vi "ServerProcess.vi"(0 "occurrence":refnum<k4>, 1 "TCP port":u16=62001, 5 "error in (no error)":errorcluster) -> (19 "error out":errorcluster)   [LabVIEW 2017, in "G#DebugServer.lvclass"]
doc: "Server process on the remote target."
uses:
  G#DebugServer.lvclass
  utils/LocalProcessData.ctl
  utils/TCPCommand.ctl
  G#Object/utils/G#Object_Event.ctl
  G#Object/utils/G#Object_EventType.ctl
  G#Object/utils/G#Object_ObjectInfoType.ctl
  G#Object/utils/G#Object_CreateMethod.ctl
  G#Object/G#Object.lvclass
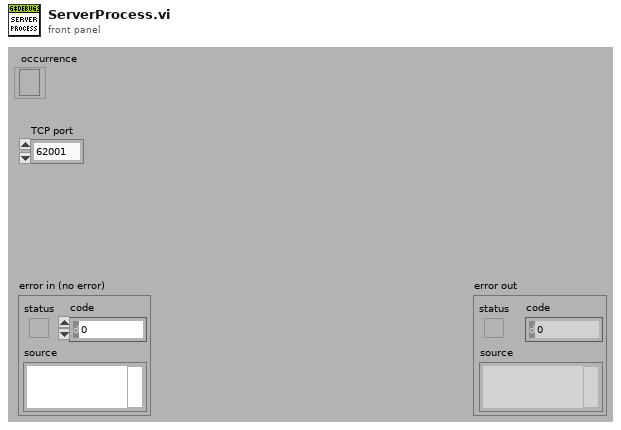
[diagram p1: front panel]
types:
  T1 = cluster{"ClientAddress":u32, "G#Event":refnum<user-event>, "CreatedG#event?":bool, "ConnectionID":refnum<k5>, "Enabled":bool}
  T2 = typedef "G#Object.lvclass/G#Object_Event.ctl" = cluster{"EventType":T3, "ObjectInfo":T4, "Ref":refnum<class "G#Object.lvclass">, "Time Stamp":timestamp, "LogText":string, "Parameters":variant[]}
  T3 = typedef "G#Object.lvclass/G#Object_EventType.ctl" = enum16{"Created new", "Looked up existing", "Deleted", "Forced delete", "Not deleted", "Garbage collected", "Cleared", "User", "Error", "External create object", "External create class attributes", "Created class attributes", "Run constructor", "Run constructor done", "Run open method", "Run open method done"}
  T4 = typedef "G#Object.lvclass/G#Object_ObjectInfoType.ctl" = cluster{"ObjectName":string, "ObjectID":u32, "Users":i32, "Counter":bool, "AttributeRefs":u32[], "FullClassName":string, "ClassName":string, "CreateMethod":T5, "GenericDestructorExists":bool, "Owner":string}
  T5 = typedef "G#Object.lvclass/G#Object_CreateMethod.ctl" = enum16{"Create", "Create or look up existing", "Look up existing"}
  T6 = typedef "G#DebugServer.lvclass/LocalProcessData.ctl" = cluster{"Event":string, "Command":T7, "Data":string, "Address":u32}
  T7 = typedef "G#DebugServer.lvclass/TCPCommand.ctl" = u8
  T8 = typedef "G#Object.lvclass/G#Object_ClassHierarchy.ctl" = cluster{"ClassName":string, "FullClassName":string, "ClassPath":path, "IsLeaf":bool}
  T9 = typedef "G#Object.lvclass/G#Object_ClassInfoType.ctl" = cluster{"ClassName":string, "ObjectInfo":T4[], "ObjectRefs":refnum<class "G#Object.lvclass">[], "TypeRef":refnum<class "G#Object.lvclass">}
  T10 = cluster{"G#DebugServer ref":refnum<class "G#Object.lvclass">, "attributes":variant[]}
  T11 = cluster{"G#DebugServer ref":refnum<class "G#Object.lvclass">, "class attributes":variant[]}
  T12 = cluster{"G#DebugServer ref":refnum<class "G#Object.lvclass">, "string":string}
  T13 = cluster{"G#DebugServer ref":refnum<class "G#Object.lvclass">, "class hierarchy":T8[]}
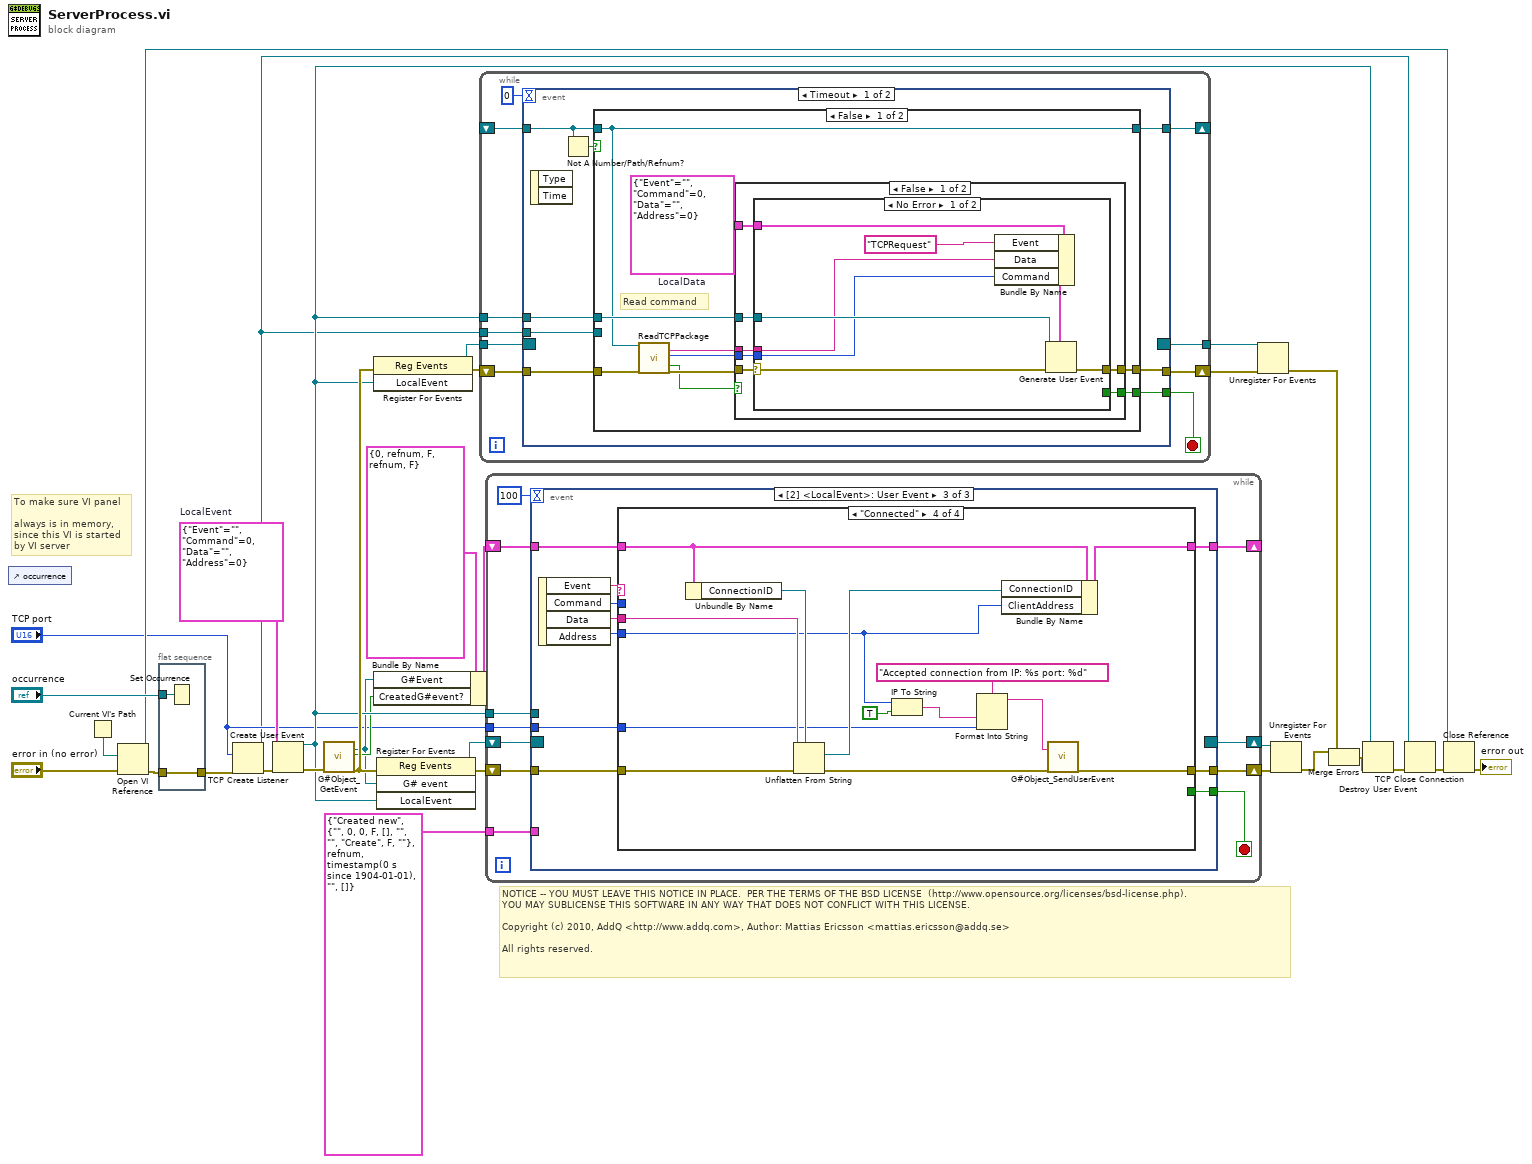
[diagram p0: block diagram]
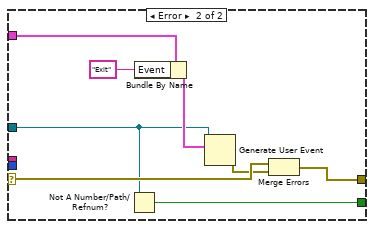
[diagram p2: hidden frame]
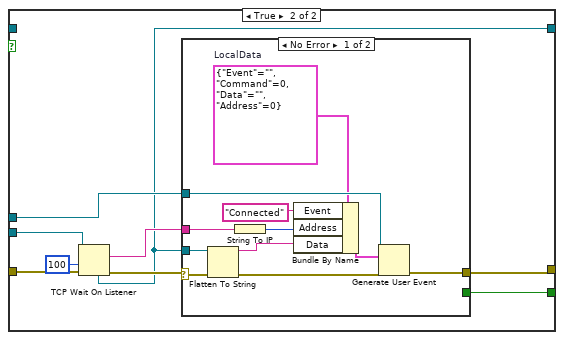
[diagram p4: hidden frame]
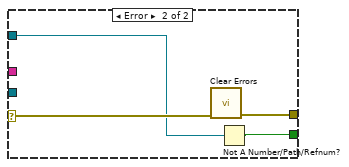
[diagram p5: hidden frame]
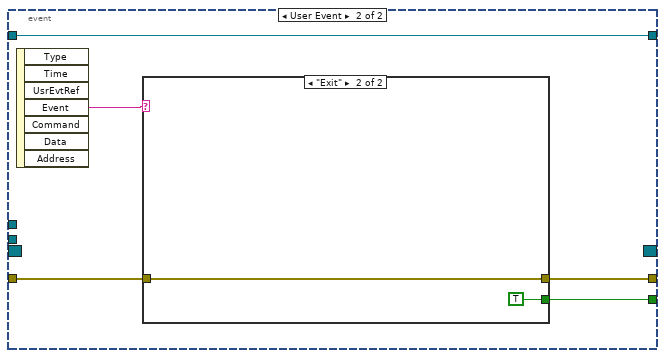
[diagram p6: hidden frame]
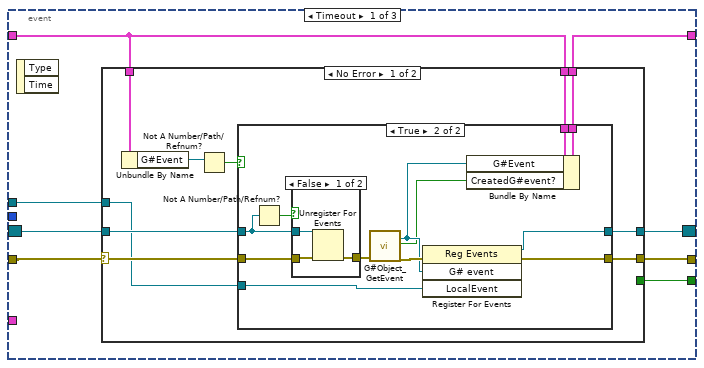
[diagram p8: hidden frame]
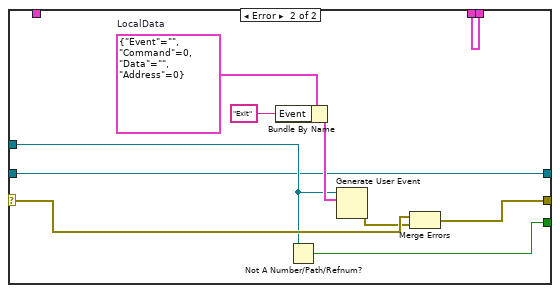
[diagram p11: hidden frame]
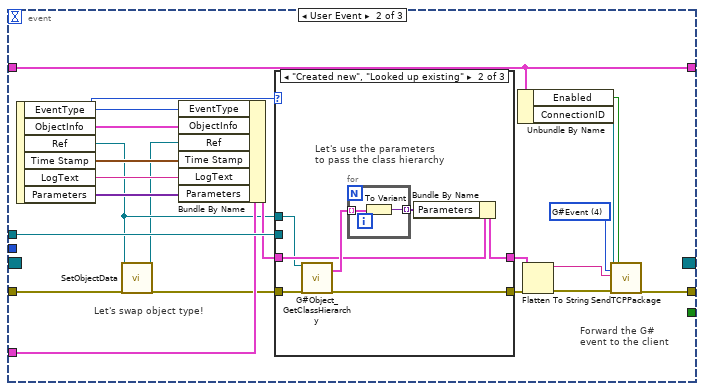
[diagram p12: hidden frame]
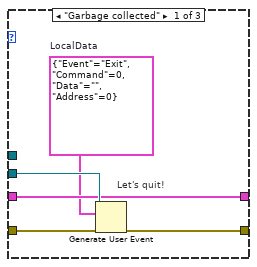
[diagram p13: hidden frame]
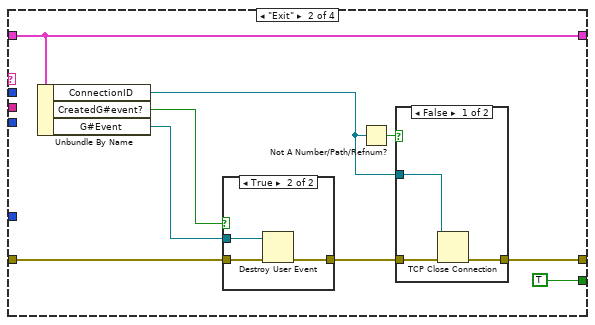
[diagram p16: hidden frame]
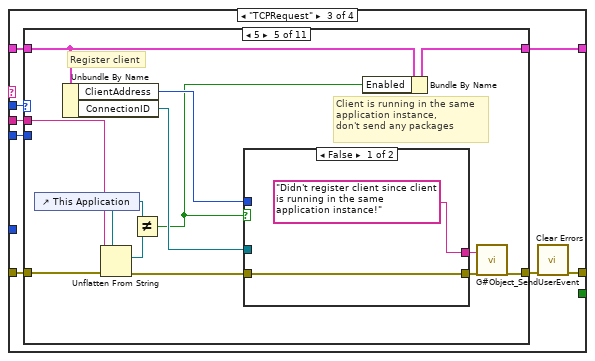
[diagram p19: hidden frame]
diagram:
  w13 = T6 {"Event"="", "Command"=0, "Data"="", "Address"=0}  # LocalEvent
  # "NOTICE -- YOU MUST LEAVE THIS NOTICE IN PLACE.  PER THE TERMS OF THE BSD LICENSE  (http://www.opensource.org/licenses/bsd-license.php).\nYOU MAY SUBLICENSE THIS SOFTWARE IN ANY WAY THAT DOES NOT CONFLICT WITH THIS LICENSE.\n\nCopyright (c) 2010, AddQ <http://www.addq.com>, Author: Mattias Ericsson <mattias.ericsson@addq.se>\n\nAll rights reserved."
  # "To make sure VI panel\n\nalways is in memory,\nsince this VI is started\nby VI server"
  n1 = control-ref of="occurrence"() -> ()  [unwired: 1 out]
  n2 = Current VI's Path() -> (path=w32:path)
  n3 = Open VI Reference(vi path=w32, error in (no error)="error in (no error)") -> (vi reference=w27:refnum<vi>, error out=w30:errorcluster)  [unwired: 4 in]
  n4 = flat-sequence {
    tunnel: "occurrence" -> [w34]
    tunnel: w30 -> [w33]
    tunnel: [w33] -> w6
    frame #0 {
      n5 = Set Occurrence(w34) -> ()
    }
  }
  n6 = TCP Create Listener(8:w6, 10:"TCP port") -> (0:w5:errorcluster, 3:w1:refnum<k5>)  [unwired: 3 in, 1 out]
  n7 = Create User Event(user event datatype=w13, error in=w5) -> (user event=w12:refnum<user-event>, error out=w15:errorcluster)
  n8 = call "G#Object_GetEvent.vi"("error in (no error)"=w15) -> ("G# event"=w7:refnum<user-event>, "created new"=w8:bool, "error out"=w14:errorcluster)  [unwired: 14 in, 2 out]
  n9 = register-events(error in=w14, w12) -> (reference out=w17:refnum<event-registration>, error out=w22:errorcluster)  [unwired: 1 in]
  n10 = Bundle By Name(cluster=T1 {"ClientAddress"=0, "G#Event"=refnum, "CreatedG#event?"=FALSE, "ConnectionID"=refnum, "Enabled"=FALSE}, "G#Event"=w7, "CreatedG#event?"=w8) -> (w9:T1)
  n11 = register-events(error in=w14, w7, w12) -> (reference out=w25:refnum<event-registration>, error out=w26:errorcluster)  [unwired: 1 in]
  n12 = while {
    shift-right: [w41] -> w21
    shift-left: w22 -> [w42]
    tunnel: [w44] -> w20
    tunnel: w17 -> [w43]
    tunnel: w1 -> [w40]
    tunnel: w12 -> [w37]
    shift-right: [w36] -> _
    shift-left: _ -> [w35]
    stop <- w39 stop-if-true
    n13 = event shown="[0] Timeout" {
      selector: w43 -> [_ _]
      dyn-events: [_ _] -> w44
      timeout: 0 -> [_ _]
      tunnel: w42 -> [w50 w115]
      tunnel: [w51 w114] -> w41
      tunnel: w40 -> [w48 _]
      tunnel: [w49 w113] -> w39
      tunnel: w37 -> [w52 _]
      tunnel: [w47 w111] -> w36
      tunnel: w35 -> [w45 w111]
      event Timeout {
        n14 = event-data() -> ()  [unwired: 1 in, 2 out]
        n15 = Not A Number/Path/Refnum?(number/path/refnum=w45) -> (NaN/Path/Refnum?=w46:bool)
        n16 = case shown="False" w46 {
          tunnel: w52 -> [w62 w90]
          tunnel: [w61 w92] -> w51
          tunnel: w50 -> [w59 w95]
          tunnel: [w54 w89] -> w49
          tunnel: w48 -> [_ w94]
          tunnel: [w53 w87] -> w47
          tunnel: w45 -> [w53 _]
          frame False {
            w60 = T6 {"Event"="", "Command"=0, "Data"="", "Address"=0}  # LocalData
            # "Read command"
            n17 = call "ReadTCPPackage.vi"("connection ID"=w53, "error in (no error)"=w59) -> ("payload"=w56:string, "command"=w55:T7, "timeout"=w57:bool, "error out"=w58:errorcluster)  [unwired: 14 in]
            n18 = case shown="False" w57 {
              tunnel: w58 -> [w69 w86]
              tunnel: [w67 w86] -> w61
              tunnel: w62 -> [w68 _]
              tunnel: w60 -> [w66 _]
              tunnel: w56 -> [w65 _]
              tunnel: w55 -> [w64 _]
              tunnel: [w63 _] -> w54
              frame False {
                n19 = case shown="No Error" w69 {
                  selector: w69 -> [w72 w84]
                  tunnel: w68 -> [w77 w79]
                  tunnel: [w76 w85] -> w67
                  tunnel: w66 -> [w75 w82]
                  tunnel: w65 -> [w71 _]
                  tunnel: w64 -> [w70 _]
                  tunnel: [_ w78] -> w63
                  frame No Error {
                    n20 = Bundle By Name(cluster=w75, "Event"="TCPRequest" ("Command"), "Data"=w71, "Command"=w70) -> (w74:T6)
                    n21 = Generate User Event(user event=w77, event data cluster=w74, error in=w72) -> (error out=w76:errorcluster)  [unwired: 1 in, 1 out]
                  }
                  frame Error {
                    n22 = Not A Number/Path/Refnum?(number/path/refnum=w79) -> (NaN/Path/Refnum?=w78:bool)
                    n23 = Bundle By Name(cluster=w82, "Event"="Exit" ("Command")) -> (w81:T6)
                    n24 = Generate User Event(user event=w79, event data cluster=w81) -> (error out=w83:errorcluster)  [unwired: 2 in, 1 out]
                    n25 = Merge Errors(w84, w83) -> (w85:errorcluster)
                  }
                }
              }
              frame True {
                # "Timeout"
              }
            }
          }
          frame True {
            n26 = TCP Wait On Listener(8:w95, 9:100 ("timeout ms (wait forever: -1)"), 11:w94) -> (0:w91:errorcluster, 2:w88:string, 4:w87:refnum<k5>)  [unwired: 1 in, 2 out]
            n27 = case shown="No Error" w91 {
              selector: w91 -> [w100 w109]
              tunnel: [w106 w110] -> w92
              tunnel: w90 -> [w105 w108]
              tunnel: [_ w107] -> w89
              tunnel: w88 -> [w101 _]
              tunnel: w87 -> [w98 _]
              frame No Error {
                w104 = T6 {"Event"="", "Command"=0, "Data"="", "Address"=0}  # LocalData
                n28 = Flatten To String(anything=w98, error in (no error)=w100) -> (data string=w97:string, error out=w99:errorcluster)  [unwired: 2 in, 1 out]
                n29 = String To IP(1:w101) -> (0:w102:u32)
                n30 = Bundle By Name(cluster=w104, "Event"="Connected", "Address"=w102, "Data"=w97) -> (w103:T6)
                n31 = Generate User Event(user event=w105, event data cluster=w103, error in=w99) -> (error out=w106:errorcluster)  [unwired: 1 in, 1 out]
              }
              frame Error {
                n32 = call <vilib>:"Clear Errors.vi"("error in (no error)"=w109) -> ("error out"=w110:errorcluster)  [unwired: 5 in, 1 out]
                n33 = Not A Number/Path/Refnum?(number/path/refnum=w108) -> (NaN/Path/Refnum?=w107:bool)
              }
            }
          }
        }
      }
      event User Event {
        n34 = event-data() -> ("Event"=w112:string)  [unwired: 1 in, 6 out]
        n35 = case shown="\"Exit\"" w112 {
          tunnel: w115 -> [w116 w117]
          tunnel: [w116 w117] -> w114
          tunnel: [_ TRUE] -> w113
          frame Default {
          }
          frame "Exit" {
          }
        }
      }
    }
  }
  n36 = while {
    shift-right: [w126] -> w24
    shift-left: w26 -> [w127]
    tunnel: w12 -> [w124]
    tunnel: T2 {"EventType"=enum."Created new", "ObjectInfo"={"ObjectName"="", "ObjectID"=0, "Users"=0, "Counter"=FALSE, "AttributeRefs"=[], "FullClassName"="", "ClassName"="", "CreateMethod"=enum."Create", "GenericDestructorExists"=FALSE, "Owner"=""}, "Ref"=refnum, "Time Stamp"=timestamp(0 s since 1904-01-01), "LogText"="", "Parameters"=[]} ("G#Event") -> [w122]
    shift-right: [w121] -> _
    shift-left: w9 -> [w120]
    shift-right: [w128] -> w23
    shift-left: w25 -> [w129]
    tunnel: "TCP port" -> [w119]
    stop <- w125 stop-if-true
    n37 = event shown="[2] <LocalEvent>: User Event" {
      selector: w129 -> [w133 _ _]
      dyn-events: [w132 _ _] -> w128
      timeout: 100 -> [_ _ _]
      tunnel: [w135 w179 w221] -> w126
      tunnel: w127 -> [w137 w184 w223]
      tunnel: [w134 _ w220] -> w125
      tunnel: w124 -> [w136 w197 _]
      tunnel: w122 -> [_ w192 _]
      tunnel: [w130 w180 w216] -> w121
      tunnel: w120 -> [w131 w180 w215]
      tunnel: w119 -> [_ _ w214]
      event Timeout {
        n38 = event-data() -> ()  [unwired: 1 in, 2 out]
        n39 = case shown="No Error" w137 {
          selector: w137 -> [w145 w175]
          tunnel: w136 -> [w142 w171]
          tunnel: [w141 w176] -> w135
          tunnel: [_ w170] -> w134
          tunnel: w133 -> [w146 w167]
          tunnel: w131 -> [w144 _]
          tunnel: [w140 w167] -> w132
          tunnel: w131 -> [w139 w168]
          tunnel: [w138 w168] -> w130
          frame No Error {
            n40 = Unbundle By Name(w144) -> ("G#Event"=w143:refnum<user-event>)
            n41 = Not A Number/Path/Refnum?(number/path/refnum=w143) -> (NaN/Path/Refnum?=w147:bool)
            n42 = case shown="True" w147 {
              tunnel: w146 -> [w148 w160]
              tunnel: w145 -> [w149 w161]
              tunnel: w142 -> [_ w157]
              tunnel: [w149 w156] -> w141
              tunnel: [w148 w155] -> w140
              tunnel: w139 -> [w150 w154]
              tunnel: [w150 w153] -> w138
              frame False {
              }
              frame True {
                n43 = Not A Number/Path/Refnum?(number/path/refnum=w160) -> (NaN/Path/Refnum?=w162:bool)
                n44 = case shown="False" w162 {
                  tunnel: w161 -> [w165 w166]
                  tunnel: w160 -> [w164 _]
                  tunnel: [w163 w166] -> w159
                  frame False {
                    n45 = Unregister For Events(event registration refnum=w164, error in=w165) -> (error out=w163:errorcluster)
                  }
                  frame True {
                  }
                }
                n46 = call "G#Object_GetEvent.vi"("error in (no error)"=w159) -> ("G# event"=w152:refnum<user-event>, "created new"=w151:bool, "error out"=w158:errorcluster)  [unwired: 14 in, 2 out]
                n47 = register-events(error in=w158, w152, w157) -> (reference out=w155:refnum<event-registration>, error out=w156:errorcluster)  [unwired: 1 in]
                n48 = Bundle By Name(cluster=w154, "G#Event"=w152, "CreatedG#event?"=w151) -> (w153:T1)
              }
            }
          }
          frame Error {
            w169 = T6 {"Event"="", "Command"=0, "Data"="", "Address"=0}  # LocalData
            n49 = Bundle By Name(cluster=w169, "Event"="Exit" ("Command")) -> (w172:T6)
            n50 = Not A Number/Path/Refnum?(number/path/refnum=w171) -> (NaN/Path/Refnum?=w170:bool)
            n51 = Generate User Event(user event=w171, event data cluster=w172) -> (error out=w174:errorcluster)  [unwired: 2 in, 1 out]
            n52 = Merge Errors(w175, w174) -> (w176:errorcluster)
          }
        }
      }
      event User Event {
        w189 = T7 4 items=["GarbageCollect", "GetAllObjects", "GetAllObjectsReply", "CleanUp", "G#Event"] ("Command")
        # "Let's swap object type!"
        # "Forward the G#\nevent to the client"
        n53 = event-data() -> ("EventType"=w196:T3, "ObjectInfo"=w195:T4, "Ref"=w182:refnum<class "G#Object.lvclass">, "Time Stamp"=w194:timestamp, "LogText"=w193:string, "Parameters"=w190:variant[])  [unwired: 1 in]
        n54 = call "SetObjectData.vi"("real object ref"=w182, "error in (no error)"=w184) -> ("remote ref"=w181:refnum<class "G#Object.lvclass">, "error out"=w183:errorcluster)  [unwired: 16 in]
        n55 = Bundle By Name(cluster=w192, "EventType"=w196, "ObjectInfo"=w195, "Ref"=w181, "Time Stamp"=w194, "LogText"=w193, "Parameters"=w190) -> (w191:T2)
        n56 = case shown="\"Created new\", \"Looked up existing\"" w196 {
          tunnel: w183 -> [w202 w209 w213]
          tunnel: [w201 w208 w213] -> w186
          tunnel: w197 -> [w200 _ _]
          tunnel: w191 -> [w199 w206 w212]
          tunnel: [w199 w205 w212] -> w185
          tunnel: w182 -> [_ w204 _]
          frame "Garbage collected" {
            w198 = T6 {"Event"="Exit", "Command"=0, "Data"="", "Address"=0}  # LocalData
            # "Let's quit!"
            n57 = Generate User Event(user event=w200, event data cluster=w198, error in=w202) -> (error out=w201:errorcluster)  [unwired: 1 in, 1 out]
          }
          frame "Created new", "Looked up existing" {
            # "Let's use the parameters\nto pass the class hierarchy"
            n58 = call "G#Object_GetClassHierarchy.vi"("reference in"=w204, "error in (no error)"=w209) -> ("class hierarchy"=w207:T8[], "error out"=w208:errorcluster)  [unwired: 15 in, 1 out]
            n59 = for {
              tunnel: w207 -> [w211] mode=indexing
              tunnel: [w210] -> w203 mode=indexing
              n60 = To Variant(anything=w211) -> (Variant=w210:variant)
            }
            n61 = Bundle By Name(cluster=w206, "Parameters"=w203) -> (w205:T2)
          }
          frame Default {
          }
        }
        n62 = Unbundle By Name(w180) -> ("Enabled"=w177:bool, "ConnectionID"=w178:refnum<k5>)
        n63 = Flatten To String(anything=w185, error in (no error)=w186) -> (data string=w187:string, error out=w188:errorcluster)  [unwired: 2 in, 1 out]
        n64 = call "SendTCPPackage.vi"("connection ID"=w178, "command"=w189, "data"=w187, "error in (no error)"=w188, "enabled"=w177) -> ("error out"=w179:errorcluster)  [unwired: 14 in]
      }
      event User Event {
        n65 = event-data() -> ("Event"=w222:string, "Command"=w219:T7, "Data"=w218:string, "Address"=w217:u32)  [unwired: 1 in]
        n66 = case shown="\"Connected\"" w222 {
          tunnel: w223 -> [w225 w233 w249 w476]
          tunnel: [w225 w227 w243 w465] -> w221
          tunnel: [_ TRUE _ _] -> w220
          tunnel: w219 -> [_ _ w250 _]
          tunnel: w218 -> [_ _ w248 w475]
          tunnel: w217 -> [_ _ w247 w467]
          tunnel: [w224 w232 w246 w472] -> w216
          tunnel: w215 -> [w224 w232 w245 w473]
          tunnel: w214 -> [_ _ _ w463]
          frame Default {
          }
          frame "Exit" {
            n67 = Unbundle By Name(w232) -> ("ConnectionID"=w226:refnum<k5>, "CreatedG#event?"=w231:bool, "G#Event"=w230:refnum<user-event>)
            n68 = case shown="True" w231 {
              tunnel: w233 -> [w239 w242]
              tunnel: [w239 w241] -> w228
              tunnel: w230 -> [_ w240]
              frame False {
              }
              frame True {
                n69 = Destroy User Event(user event=w240, error in=w242) -> (error out=w241:errorcluster)
              }
            }
            n70 = Not A Number/Path/Refnum?(number/path/refnum=w226) -> (NaN/Path/Refnum?=w229:bool)
            n71 = case shown="False" w229 {
              tunnel: w228 -> [w237 w238]
              tunnel: [w236 w238] -> w227
              tunnel: w226 -> [w235 _]
              frame False {
                n72 = TCP Close Connection(connection ID=w235, error in (no error)=w237) -> (error out=w236:errorcluster)  [unwired: 1 in, 1 out]
              }
              frame True {
              }
            }
          }
          frame "TCPRequest" {
            n73 = case shown="5" w250 {
              tunnel: w249 -> [w252 w256 w268 w287 w300 w317 w364 w402 w425 w445 w454]
              tunnel: [w252 w255 w266 w286 w295 w322 w368 w406 w429 w441 w455] -> w244
              tunnel: w248 -> [_ _ _ _ w299 w316 w363 w401 w422 w444 _]
              tunnel: w247 -> [_ _ _ _ _ _ _ _ _ _ _]
              tunnel: [w251 w253 w259 w285 w296 w313 w359 w397 w420 w446 w457] -> w246
              tunnel: w245 -> [w251 w253 w259 w285 w293 w313 w359 w397 w420 w446 w458]
              frame Default {
              }
              frame 0 {
                w254 = FALSE  # only from same owner as caller? (T)
                # "Garbage Collect"
                n74 = call "GarbageCollector.vi"("only from same owner as caller? (T)"=w254, "error in (no error)"=w256) -> ("error out"=w255:errorcluster)  [unwired: 15 in, 2 out]
              }
              frame 1 {
                w265 = T7 2 items=["GarbageCollect", "GetAllObjects", "GetAllObjectsReply", "CleanUp", "G#Event"] ("Command")
                # "Swap objects!"
                # "Get All Object"
                n75 = call "G#Object_GetAllObjects.vi"("error in (no error)"=w268) -> ("class information"=w262:T9[], "error out"=w263:errorcluster)  [unwired: 15 in, 2 out]
                n76 = for {
                  shift-right: [w278] -> w261
                  shift-left: w263 -> [w274]
                  tunnel: w262 -> [w277] mode=indexing
                  tunnel: [w269] -> w260 mode=indexing
                  n77 = Unbundle By Name(w277) -> ("ObjectRefs"=w279:refnum<class "G#Object.lvclass">[], "TypeRef"=w273:refnum<class "G#Object.lvclass">)
                  n78 = call "G#Object_GetClassHierarchy.vi"("reference in"=w273, "error in (no error)"=w274) -> ("class hierarchy"=w270:T8[], "error out"=w272:errorcluster)  [unwired: 15 in, 1 out]
                  n79 = call "SetObjectData.vi"("real object ref"=w273, "error in (no error)"=w272) -> ("remote ref"=w275:refnum<class "G#Object.lvclass">, "error out"=w280:errorcluster)  [unwired: 16 in]
                  n80 = for {
                    shift-right: [w284] -> w278
                    shift-left: w280 -> [w283]
                    tunnel: w279 -> [w282] mode=indexing
                    tunnel: [w281] -> w276 mode=indexing
                    n81 = call "SetObjectData.vi"("real object ref"=w282, "error in (no error)"=w283) -> ("remote ref"=w281:refnum<class "G#Object.lvclass">, "error out"=w284:errorcluster)  [unwired: 16 in]
                  }
                  n82 = Bundle By Name(cluster=w277, "ObjectRefs"=w276, "TypeRef"=w275) -> (w271:T9)
                  n83 = Bundle(w271, "class hierarchy"=w270) -> (w269:cluster{T9, "class hierarchy":T8[]})  [unwired: 1 in]
                }
                n84 = Unbundle By Name(w259) -> ("Enabled"=w257:bool, "ConnectionID"=w258:refnum<k5>)
                n85 = Flatten To String(anything=w260, error in (no error)=w261) -> (data string=w264:string, error out=w267:errorcluster)  [unwired: 2 in, 1 out]
                n86 = call "SendTCPPackage.vi"("connection ID"=w258, "command"=w265, "data"=w264, "error in (no error)"=w267, "enabled"=w257) -> ("error out"=w266:errorcluster)  [unwired: 14 in]
              }
              frame 3 {
                # "Clean up"
                n87 = call "G#Object_CleanUp.vi"("error in (no error)"=w287) -> ("error out"=w286:errorcluster)  [unwired: 17 in, 1 out]
              }
              frame 5 {
                # "Client is running in the same\napplication instance,\ndon't send any packages"
                # "Register client"
                n88 = control-ref of="This Application"() -> (w298:refnum<vi>)
                n89 = Unbundle By Name(w293) -> ("ClientAddress"=w289:u32, "ConnectionID"=w291:refnum<k5>)
                n90 = Unflatten From String(type=w298, binary string=w299, error in (no error)=w300) -> (value=w297:refnum<vi>, error out=w292:errorcluster)  [unwired: 2 in, 1 out]
                n91 = Not Equal?(x=w298, y=w297) -> (x != y?=w288:bool)
                n92 = case shown="False" w288 {
                  tunnel: w289 -> [_ w308]
                  tunnel: ["Didn't register client since client is running in the same application instance!" w304] -> w294
                  tunnel: w292 -> [w301 w303]
                  tunnel: w291 -> [_ _]
                  tunnel: [w301 w303] -> w290
                  frame False {
                  }
                  frame True {
                    n93 = IP To String(1:TRUE ("dot notation? (F)"), 2:w308) -> (0:w305:string)
                    n94 = Format Into String(format string="Register client IP: %s", w305) -> (resulting string=w304:string)  [unwired: 2 in, 1 out]
                  }
                }
                n95 = Bundle By Name(cluster=w293, "Enabled"=w288) -> (w296:T1)
                n96 = call "G#Object_SendUserEvent.vi"("text"=w294, "error in (no error)"=w290) -> ("error out"=w295:errorcluster)  [unwired: 16 in, 1 out]
              }
              frame 6 {
                w319 = T7 7 items=["GarbageCollect", "GetAllObjects", "GetAllObjectsReply", "CleanUp", "G#Event", "RegisterClient", "GetAttributeValue", "GetAttributeValueReply", "GetClassAttributeValue", "GetClassAttributeValueReply"] ("Command")
                # "GetAttributeValue"
                n97 = Unbundle By Name(w313) -> ("Enabled"=w309:bool, "ConnectionID"=w310:refnum<k5>)
                n98 = call "FindRealObject.vi"("flattened remote ref"=w316, "error in (no error)"=w317) -> ("G#DebugServer ref"=w314:refnum<class "G#Object.lvclass">, "real object ref"=w315:refnum<class "G#Object.lvclass">, "not found"=w312:bool, "in client memory?"=w311:bool, "error out"=w318:errorcluster)  [unwired: 13 in]
                n99 = case shown="False" w312 {
                  tunnel: [w323 w354] -> w321
                  tunnel: [w324 ""] -> w320
                  tunnel: w318 -> [w331 w354]
                  tunnel: w315 -> [w330 _]
                  tunnel: w314 -> [w328 _]
                  tunnel: w311 -> [w329 _]
                  frame False {
                    n100 = call "G#Object_GetAttributeValue.vi"("reference in"=w330, "error in (no error)"=w331) -> ("attributes"=w325:variant[], "valid object"=w326:bool, "error out"=w327:errorcluster)  [unwired: 13 in, 2 out]
                    n101 = case shown="True" w326 {
                      tunnel: w327 -> [w333 w338]
                      tunnel: [w333 w342] -> w323
                      tunnel: ["" w341] -> w324
                      tunnel: w325 -> [_ w336]
                      tunnel: w328 -> [_ w340]
                      tunnel: w329 -> [_ w334]
                      frame False {
                      }
                      frame True {
                        n102 = case shown="False" w334 {
                          tunnel: w338 -> [w346 w351]
                          tunnel: [w345 w351] -> w337
                          tunnel: w336 -> [w344 w352]
                          tunnel: [w343 w352] -> w335
                          frame False {
                            n103 = for {
                              tunnel: w344 -> [w348] mode=indexing
                              tunnel: [w347] -> w343 mode=indexing
                              shift-right: [w349] -> w345
                              shift-left: w346 -> [w350]
                              n104 = call "ReplaceClassReferences.vi"("attribute data"=w348, "error in (no error)"=w350) -> ("attribute data out"=w347:variant, "error out"=w349:errorcluster)  [unwired: 16 in]
                            }
                          }
                          frame True {
                          }
                        }
                        n105 = Bundle("G#DebugServer ref"=w340, "attributes"=w335) -> (w339:T10)  [unwired: 1 in]
                        n106 = Flatten To String(anything=w339, error in (no error)=w337) -> (data string=w341:string, error out=w342:errorcluster)  [unwired: 2 in, 1 out]
                      }
                    }
                  }
                  frame True {
                  }
                }
                n107 = call "SendTCPPackage.vi"("connection ID"=w310, "command"=w319, "data"=w320, "error in (no error)"=w321, "enabled"=w309) -> ("error out"=w322:errorcluster)  [unwired: 14 in]
              }
              frame 8 {
                w365 = T7 9 items=["GarbageCollect", "GetAllObjects", "GetAllObjectsReply", "CleanUp", "G#Event", "RegisterClient", "GetAttributeValue", "GetAttributeValueReply", "GetClassAttributeValue", "GetClassAttributeValueReply"] ("Command")
                # "GetClassAttributeValue"
                n108 = call "FindRealClassTypeObject.vi"("flattened remote ref"=w363, "error in (no error)"=w364) -> ("G#DebugServer ref"=w362:refnum<class "G#Object.lvclass">, "real ibject ref"=w361:refnum<class "G#Object.lvclass">, "not found?"=w358:bool, "in host memory?"=w357:bool, "error out"=w360:errorcluster)  [unwired: 13 in]
                n109 = case shown="False" w358 {
                  tunnel: [w380 w393] -> w367
                  tunnel: [w379 ""] -> w366
                  tunnel: w362 -> [w373 _]
                  tunnel: w361 -> [w376 _]
                  tunnel: w360 -> [w375 w393]
                  tunnel: w357 -> [w372 _]
                  frame False {
                    n110 = call "G#Object_GetAttributeValue.vi"("reference in"=w376, "object attributes (T)"=FALSE, "class attributes (F)"=TRUE, "error in (no error)"=w375) -> ("class attributes"=w374:variant[], "error out"=w381:errorcluster)  [unwired: 11 in, 3 out]
                    n111 = case shown="False" w372 {
                      tunnel: w381 -> [w385 w390]
                      tunnel: [w384 w390] -> w370
                      tunnel: w374 -> [w383 w391]
                      tunnel: [w382 w391] -> w369
                      frame False {
                        n112 = for {
                          tunnel: w383 -> [w387] mode=indexing
                          tunnel: [w386] -> w382 mode=indexing
                          shift-right: [w388] -> w384
                          shift-left: w385 -> [w389]
                          n113 = call "ReplaceClassReferences.vi"("attribute data"=w387, "error in (no error)"=w389) -> ("attribute data out"=w386:variant, "error out"=w388:errorcluster)  [unwired: 16 in]
                        }
                      }
                      frame True {
                      }
                    }
                    n114 = Bundle("G#DebugServer ref"=w373, "class attributes"=w369) -> (w371:T11)  [unwired: 1 in]
                    n115 = Flatten To String(anything=w371, error in (no error)=w370) -> (data string=w379:string, error out=w380:errorcluster)  [unwired: 2 in, 1 out]
                  }
                  frame True {
                  }
                }
                n116 = Unbundle By Name(w359) -> ("Enabled"=w355:bool, "ConnectionID"=w356:refnum<k5>)
                n117 = call "SendTCPPackage.vi"("connection ID"=w356, "command"=w365, "data"=w366, "error in (no error)"=w367, "enabled"=w355) -> ("error out"=w368:errorcluster)  [unwired: 14 in]
              }
              frame 10 {
                w405 = T7 11 items=["GarbageCollect", "GetAllObjects", "GetAllObjectsReply", "CleanUp", "G#Event", "RegisterClient", "GetAttributeValue", "GetAttributeValueReply", "GetClassAttributeValue", "GetClassAttributeValueReply", "GetToStringValue", "GetToStringValueReply"] ("Command")
                # "Get ToString value"
                n118 = call "FindRealObject.vi"("flattened remote ref"=w401, "error in (no error)"=w402) -> ("G#DebugServer ref"=w400:refnum<class "G#Object.lvclass">, "real object ref"=w403:refnum<class "G#Object.lvclass">, "not found"=w396:bool, "error out"=w404:errorcluster)  [unwired: 13 in, 1 out]
                n119 = case shown="False" w396 {
                  tunnel: w404 -> [w414 w416]
                  tunnel: w403 -> [w413 _]
                  tunnel: w400 -> [w412 _]
                  tunnel: [w409 w416] -> w399
                  tunnel: [w407 ""] -> w398
                  frame False {
                    n120 = call-dynamic "ToString.vi"("reference in"=w413, "error in (no error)"=w414) -> ("string"=w411:string, "error out"=w410:errorcluster)  [unwired: 15 in, 1 out]
                    n121 = Bundle("G#DebugServer ref"=w412, "string"=w411) -> (w408:T12)  [unwired: 1 in]
                    n122 = Flatten To String(anything=w408, error in (no error)=w410) -> (data string=w407:string, error out=w409:errorcluster)  [unwired: 2 in, 1 out]
                  }
                  frame True {
                  }
                }
                n123 = Unbundle By Name(w397) -> ("Enabled"=w394:bool, "ConnectionID"=w395:refnum<k5>)
                n124 = call "SendTCPPackage.vi"("connection ID"=w395, "command"=w405, "data"=w398, "error in (no error)"=w399, "enabled"=w394) -> ("error out"=w406:errorcluster)  [unwired: 14 in]
              }
              frame 12 {
                w428 = T7 13 items=["GarbageCollect", "GetAllObjects", "GetAllObjectsReply", "CleanUp", "G#Event", "RegisterClient", "GetAttributeValue", "GetAttributeValueReply", "GetClassAttributeValue", "GetClassAttributeValueReply", "GetToStringValue", "GetToStringValueReply", "GetClassHierarchy", "GetClassHierarchyReply"] ("Command")
                n125 = call "FindRealObject.vi"("flattened remote ref"=w422, "error in (no error)"=w425) -> ("G#DebugServer ref"=w421:refnum<class "G#Object.lvclass">, "real object ref"=w423:refnum<class "G#Object.lvclass">, "not found"=w419:bool, "error out"=w424:errorcluster)  [unwired: 13 in, 1 out]
                n126 = case shown="False" w419 {
                  tunnel: [w436 w439] -> w427
                  tunnel: [w435 ""] -> w426
                  tunnel: w424 -> [w434 w439]
                  tunnel: w423 -> [w433 _]
                  tunnel: w421 -> [w430 _]
                  frame False {
                    n127 = call "G#Object_GetClassHierarchy.vi"("reference in"=w433, "error in (no error)"=w434) -> ("class hierarchy"=w431:T8[], "error out"=w437:errorcluster)  [unwired: 15 in, 1 out]
                    n128 = Bundle("G#DebugServer ref"=w430, "class hierarchy"=w431) -> (w432:T13)  [unwired: 1 in]
                    n129 = Flatten To String(anything=w432, error in (no error)=w437) -> (data string=w435:string, error out=w436:errorcluster)  [unwired: 2 in, 1 out]
                  }
                  frame True {
                  }
                }
                n130 = Unbundle By Name(w420) -> ("Enabled"=w417:bool, "ConnectionID"=w418:refnum<k5>)
                n131 = call "SendTCPPackage.vi"("connection ID"=w418, "command"=w428, "data"=w426, "error in (no error)"=w427, "enabled"=w417) -> ("error out"=w429:errorcluster)  [unwired: 14 in]
              }
              frame 14 {
                # "Destroy"
                n132 = call "FindRealObject.vi"("flattened remote ref"=w444, "error in (no error)"=w445) -> ("real object ref"=w442:refnum<class "G#Object.lvclass">, "not found"=w440:bool, "error out"=w443:errorcluster)  [unwired: 13 in, 2 out]
                n133 = case shown="False" w440 {
                  tunnel: w443 -> [w449 w450]
                  tunnel: w442 -> [w448 _]
                  tunnel: [w447 w450] -> w441
                  frame False {
                    n134 = call-dynamic "Destroy.vi"("reference in"=w448, "error in (no error)"=w449) -> ("error out"=w447:errorcluster)  [unwired: 16 in, 1 out]
                  }
                  frame True {
                  }
                }
              }
              frame 15 {
                # "Remove Client"
                n135 = Unbundle By Name(w458) -> ("ConnectionID"=w452:refnum<k5>)
                n136 = Not A Number/Path/Refnum?(number/path/refnum=w452) -> (NaN/Path/Refnum?=w453:bool)
                n137 = case shown="False" w453 {
                  tunnel: [w461 w462] -> w455
                  tunnel: w454 -> [w460 w462]
                  tunnel: w452 -> [w459 _]
                  frame False {
                    n138 = TCP Close Connection(connection ID=w459, error in (no error)=w460) -> (error out=w461:errorcluster)  [unwired: 1 in, 1 out]
                  }
                  frame True {
                  }
                }
                n139 = Bundle By Name(cluster=w458, "ClientAddress"=u32 0, "Enabled"=FALSE) -> (w457:T1)
              }
            }
            n140 = call <vilib>:"Clear Errors.vi"("error in (no error)"=w244) -> ("error out"=w243:errorcluster)  [unwired: 5 in, 1 out]
          }
          frame "Connected" {
            n141 = Unbundle By Name(w473) -> ("ConnectionID"=w474:refnum<k5>)
            n142 = Unflatten From String(type=w474, binary string=w475, error in (no error)=w476) -> (value=w471:refnum<k5>, error out=w466:errorcluster)  [unwired: 2 in, 1 out]
            n143 = IP To String(1:TRUE ("dot notation? (F)"), 2:w467) -> (0:w468:string)
            n144 = Format Into String(format string="Accepted connection from IP: %s port: %d", w468, w463) -> (resulting string=w464:string)  [unwired: 2 in, 1 out]
            n145 = Bundle By Name(cluster=w473, "ConnectionID"=w471, "ClientAddress"=w467) -> (w472:T1)
            n146 = call "G#Object_SendUserEvent.vi"("text"=w464, "error in (no error)"=w466) -> ("error out"=w465:errorcluster)  [unwired: 16 in, 1 out]
          }
        }
      }
    }
  }
  n147 = Unregister For Events(event registration refnum=w20, error in=w21) -> (error out=w19:errorcluster)
  n148 = Unregister For Events(event registration refnum=w23, error in=w24) -> (error out=w18:errorcluster)
  n149 = Merge Errors(w19, w18) -> (w16:errorcluster)
  n150 = Destroy User Event(user event=w12, error in=w16) -> (error out=w4:errorcluster)
  n151 = TCP Close Connection(connection ID=w1, error in (no error)=w4) -> (error out=w3:errorcluster)  [unwired: 1 in, 1 out]
  n152 = Close Reference(reference=w27, error in (no error)=w3) -> (error out=→"error out":errorcluster)
